vi "Set Magnet Field.vi"(4 "Mode":T2, 6 "Axis":T1, 8 "error in (no error)":errorcluster, 9 "Target Rate (T/min)":dbl, 10 "Target Field (T)":dbl, 11 "instrument.PPMS in":refnum<class "instrument.PPMS1.lvclass">) -> (0 "error out":errorcluster, 3 "instrument.PPMS out":refnum<class "instrument.PPMS1.lvclass">)   [LabVIEW 2019, in "instrument.PPMS1.lvclass"]
uses:
  instrument.PPMS1.lvclass
  instrument.PPMS/Typedefs/PPMS.Magnet Field--cluster.ctl
  instrument.PPMS/instrument.PPMS.lvclass
  <userlib>/LevyLab/Levylab Instruments/Instrument Types/Cryostat/Typedefs/Magnet Mode--Enum.ctl
  Typedefs/PPMS1.Commands-enum.ctl
  <userlib>/LevyLab/Levylab Instruments/Instrument Types/Cryostat/Typedefs/Magnet Axis--Enum.ctl
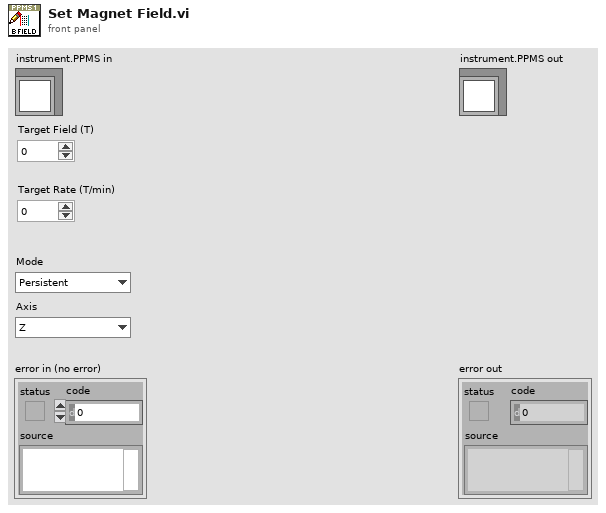
[diagram p1: front panel]
types:
  T1 = typedef "Instrument.Cryostat.lvclass/Magnet Axis--Enum.ctl" = enum16{"Z", "X", "Y"}
  T2 = typedef "Instrument.Cryostat.lvclass/Magnet Mode--Enum.ctl" = enum16{"Persistent", "Driven"}
  T3 = typedef "instrument.PPMS1.lvclass/PPMS1.Commands-enum.ctl" = enum16{"Get Magnet Field", "Get Helium Level", "Get Temperature", "Set Magnet Field", "Set Temperature", "getAll"}
  T4 = typedef "instrument.PPMS.lvclass/PPMS.Magnet Field--cluster.ctl" = cluster{"Target Field (T)":dbl, "Target Rate (T/min)":dbl, "Mode":T2}
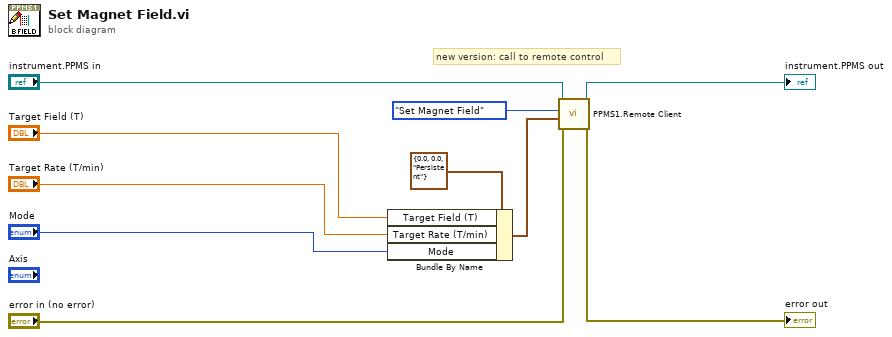
[diagram p0: block diagram]
diagram:
  # "new version: call to remote control"
  n1 = Bundle By Name(cluster=T4 {"Target Field (T)"=0.0, "Target Rate (T/min)"=0.0, "Mode"=enum."Persistent"} ("output cluster"), "Target Field (T)"="Target Field (T)", "Target Rate (T/min)"="Target Rate (T/min)", "Mode"="Mode") -> (w3:T4)
  n2 = call "PPMS1.Remote Client.vi"("error in (no error)"="error in (no error)", "Data"=w3, "Command"=PPMS1.Commands-enum."Set Magnet Field", "instrument.PPMS1 in"="instrument.PPMS in") -> ("error out"=→"error out":errorcluster, "instrument.PPMS1 out"=→"instrument.PPMS out":refnum<class "instrument.PPMS1.lvclass">)  [unwired: 4 in, 2 out]
